vi "APS set jog param.vi"(8 "error in (no error)":errorcluster caption="错误输入（无错误）", 9 "Mask":i32, 10 "pStr_Jog":T1, 11 "Axis_ID":i32) -> (0 "error out":errorcluster caption="错误输出", 2 "pStr_Jog out":T1, 3 "function return":i32)   [LabVIEW 2011, in "APS168.lvlib"]
doc: "I32 FNTYPE APS_set_jog_param( I32 Axis_ID, JOG_DATA *pStr_Jog, I32 Mask );"
uses:
  APS168.lvlib
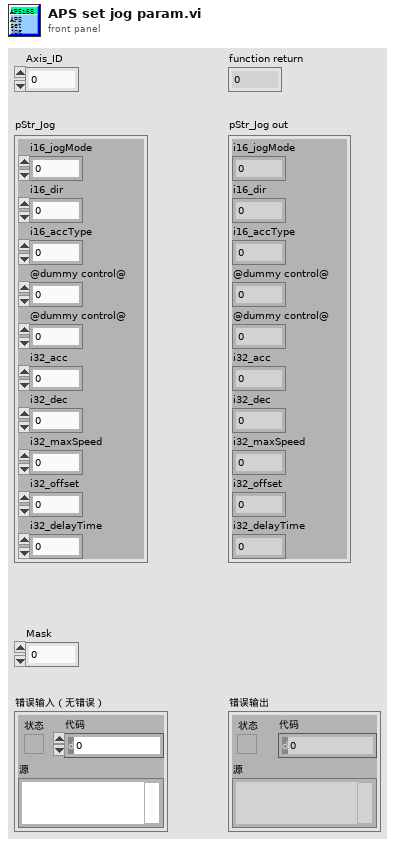
[diagram p1: front panel]
types:
  T1 = cluster{"i16_jogMode":i16, "i16_dir":i16, "i16_accType":i16, "@dummy control@":i8, "@dummy control@":i8, "i32_acc":i32, "i32_dec":i32, "i32_maxSpeed":i32, "i32_offset":i32, "i32_delayTime":i32}
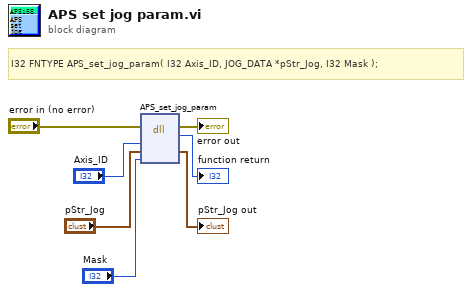
[diagram p0: block diagram]
diagram:
  # "I32 FNTYPE APS_set_jog_param( I32 Axis_ID, JOG_DATA *pStr_Jog, I32 Mask );"
  n1 = dll-call lib="PTH1Labs E软件ADLINK 204CAPS_1_7_1_LIB line 连续运动204APS168.*" fn="APS_set_jog_param"(error in="error in (no error)", "Axis_ID"="Axis_ID", "pStr_Jog"="pStr_Jog", "Mask"="Mask") -> (error out=→"error out":errorcluster, →"function return":i32, "pStr_Jog"=→"pStr_Jog out":T1)  [unwired: 4 in, 1 out]
